vi "BuildComplexClusterData.vi"(10 "Flag":bool, 11 "Array Size":i32) -> (3 "Packet":T1 {"ArrayOfClusters"."Single" format="%#.19f"; "NestedCluster"."Single" format="%#.19f"})   [LabVIEW 2015, in "MsgPack.lvlib"]
uses:
  MsgPack.lvlib
  Complex Cluster.ctl
  Simple Cluster.ctl
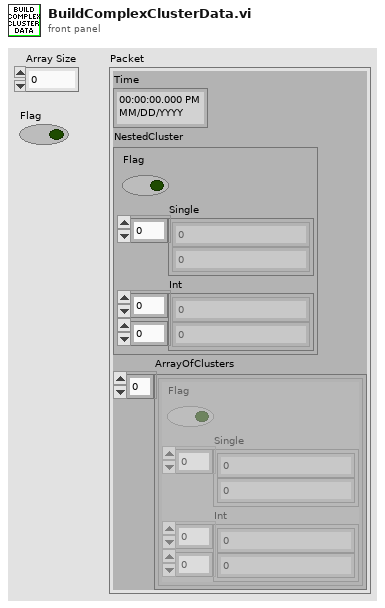
[diagram p1: front panel]
types:
  T1 = typedef "MsgPack.lvlib/Complex Cluster.ctl" = cluster{"Time":timestamp, "NestedCluster":T2, "ArrayOfClusters":T2[]}
  T2 = typedef "MsgPack.lvlib/Simple Cluster.ctl" = cluster{"Flag":bool, "Single":sgl[], "Int":i32[][]}
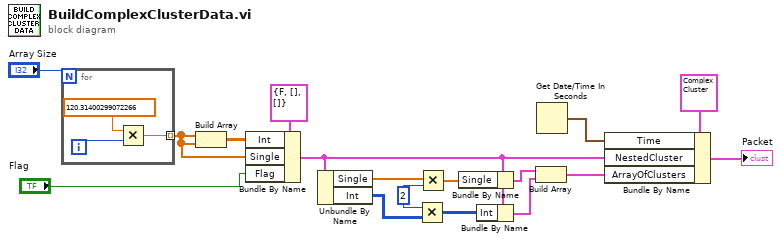
[diagram p0: block diagram]
diagram:
  w11 = 2 ("Numeric")
  n1 = for {
    N: "Array Size" -> [_]
    tunnel: [w19] -> w1 mode=indexing
    i -> [w20]
    n2 = Multiply(x=sgl 120.314, y=w20) -> (x*y=w19:sgl)
  }
  n3 = Build Array(w1, w1) -> (w2:sgl[][])
  n4 = Bundle By Name(cluster=T2 {"Flag"=FALSE, "Single"=[], "Int"=[]} ("Packet"), "Int"=w2, "Single"=w1, "Flag"="Flag") -> (w14:T2)
  n5 = Unbundle By Name(w14) -> ("Single"=w10:sgl[], "Int"=w12:i32[][])
  n6 = Multiply(x=w11, y=w12) -> (x*y=w15:i32[][])
  n7 = Multiply(x=w10, y=w11) -> (x*y=w13:sgl[])
  n8 = Bundle By Name(cluster=w14, "Single"=w13) -> (w16:T2)
  n9 = Bundle By Name(cluster=w14, "Int"=w15) -> (w17:T2)
  n10 = Build Array(w16, w17) -> (w9:T2[])
  n11 = Get Date/Time In Seconds() -> (seconds since 1Jan1904=w6:timestamp)
  n12 = Bundle By Name(cluster=T1 {"Time"=timestamp(0 s since 1904-01-01), "NestedCluster"={"Flag"=FALSE, "Single"=[], "Int"=[]}, "ArrayOfClusters"=[]} ("Packet"), "Time"=w6, "NestedCluster"=w14, "ArrayOfClusters"=w9) -> (→"Packet":T1)
